vi "Storing Random Values Into A File.vi"() -> ()   [LabVIEW 2012]
panel:
  out "String":string="Run To Select A File"
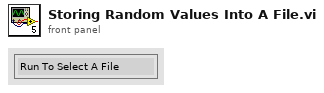
[diagram p1: front panel]
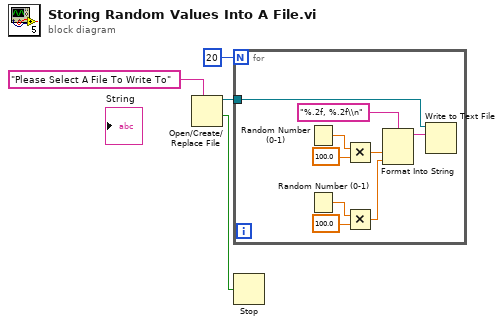
[diagram p0: block diagram]
diagram:
  n1 = Open/Create/Replace File(prompt="Please Select A File To Write To") -> (refnum out=w3:refnum<file>, cancelled=w1:bool)  [unwired: 5 in, 1 out]
  n2 = for {
    N: 20 -> [_]
    tunnel: w3 -> [w5]
    n3 = Random Number (0-1)() -> (number: 0 to 1=w13:dbl)
    n4 = Random Number (0-1)() -> (number: 0 to 1=w12:dbl)
    n5 = Multiply(x=w13, y=100.0) -> (x*y=w9:dbl)
    n6 = Multiply(x=w12, y=100.0) -> (x*y=w8:dbl)
    n7 = Format Into String(format string="%.2f, %.2f\\n", w9, w8) -> (resulting string=w6:string)  [unwired: 2 in, 1 out]
    n8 = Write to Text File(file (use dialog)=w5, text=w6) -> ()  [unwired: 2 in, 3 out]
  }
  n9 = Stop(stop? (T)=w1) -> ()
